vi "Remove UI without races.vi"(8 "error in":errorcluster, 11 "state in":T1) -> (0 "error out":errorcluster, 3 "state out":T1)   [LabVIEW 2013, in "Standard Editor.lvlib"]
uses:
  Standard Editor.lvlib
  Controls/StateCluster.ctl
  Configuration Editor/Classes/SystemConfigRepo/SystemConfigRepo.lvclass
  Configuration Editor/Classes/Systems/Systems.lvclass
  <vilib>/NI/Configuration Framework/Node/StandardEvents.ctl
  <vilib>/NI/Configuration Framework/Node/UserEventRef.ctl
  <vilib>/NI/Configuration Framework/Controls/EventCluster.ctl
  <vilib>/NI/Configuration Framework/Node/NodeChangeEvent.ctl
  <vilib>/NI/Configuration Framework/Node/NodeRef.ctl
  <vilib>/NI/Configuration Framework/Node/NISE_CEF_Node.lvclass
  <vilib>/NI/Configuration Framework/Node/CacheState.ctl
  <vilib>/NI/Configuration Framework/Node/RefreshUIEvent.ctl
  <vilib>/NI/Configuration Framework/Node/StopEvent.ctl
  <vilib>/NI/Configuration Framework/glyph manager/glyph manager.ctl
  <vilib>/picture/picture.llb/imagedata.ctl
  <vilib>/NI/AMC/Message Queue.ctl
  <vilib>/NI/AMC/Message.ctl
  <vilib>/NI/Tools/Keyed Array/KeyedArray.ctl
  <vilib>/event_ctls.llb/usereventprio.ctl
  <vilib>/NI/Configuration Framework/NISE_CEF_TreeControl.lvlib
  <vilib>/NI/Configuration Framework/glyph manager/glyph manager.lvlib
  <vilib>/NI/Tools/Keyed Array/Tools_KeyedArray.lvlib
  <vilib>/NI/AMC/AMC.lvlib
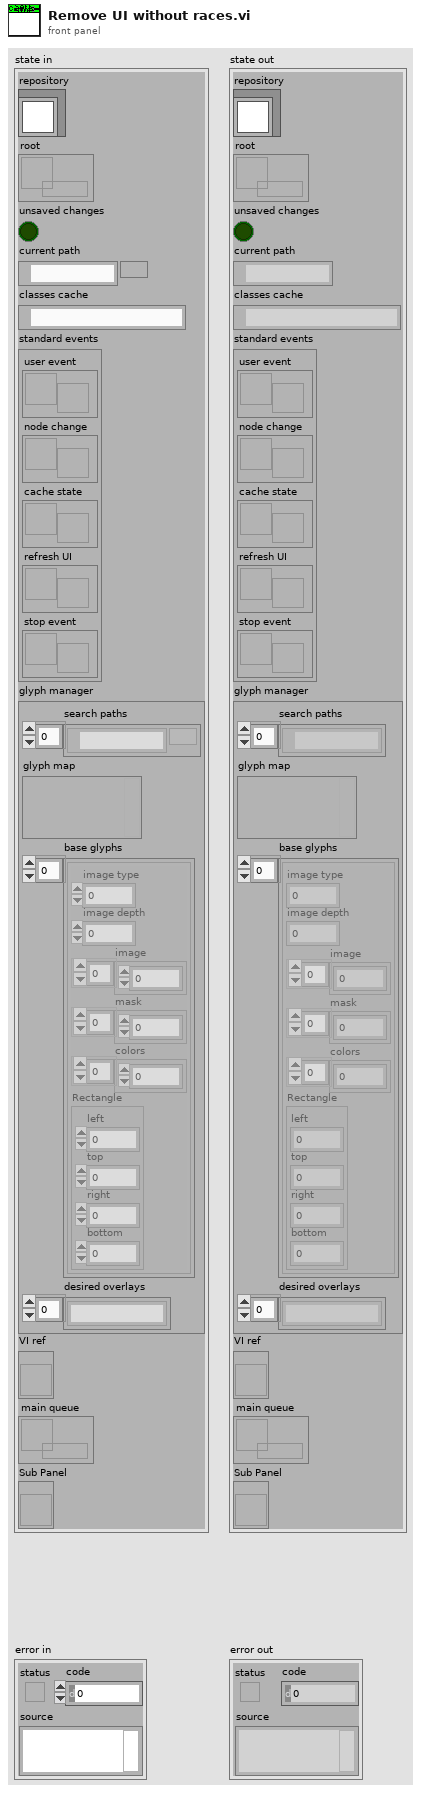
[diagram p1: front panel]
types:
  T1 = typedef "Standard Editor.lvlib/StateCluster.ctl" = cluster{"repository":refnum<class "SystemConfigRepo.lvclass">, "root":refnum<data-value>, "unsaved changes":bool, "current path":path, "classes cache":path, "standard events":T2, "glyph manager":T8, "VI ref":refnum<vi>, "main queue":T10, "Sub Panel":refnum<vi>}
  T2 = typedef "NISE_CEF_Node.lvclass/StandardEvents.ctl" = cluster{"user event":T3, "node change":T4, "cache state":T5, "refresh UI":T6, "stop event":T7}
  T3 = typedef "NISE_CEF_Node.lvclass/UserEventRef.ctl" = refnum<user-event>
  T4 = typedef "NISE_CEF_Node.lvclass/NodeChangeEvent.ctl" = refnum<user-event>
  T5 = typedef "NISE_CEF_Node.lvclass/CacheState.ctl" = refnum<user-event>
  T6 = typedef "NISE_CEF_Node.lvclass/RefreshUIEvent.ctl" = refnum<user-event>
  T7 = typedef "NISE_CEF_Node.lvclass/StopEvent.ctl" = refnum<user-event>
  T8 = typedef "glyph manager.lvlib/glyph manager.ctl" = cluster{"search paths":path[], "glyph map":variant, "base glyphs":T9[], "desired overlays":string[]}
  T9 = typedef "imagedata.ctl" = cluster{"image type":i32, "image depth":i32, "image":u8[], "mask":u8[], "colors":u32[], "Rectangle":cluster{"left":i16, "top":i16, "right":i16, "bottom":i16}}
  T10 = typedef "AMC.lvlib/Message Queue.ctl" = refnum<queue>
  T11 = typedef "usereventprio.ctl" = enum32{"high priority", "normal priority"}
  T12 = typedef "NISE_CEF_TreeControl.lvlib/EventCluster.ctl" = cluster{"command":string, "data":string}
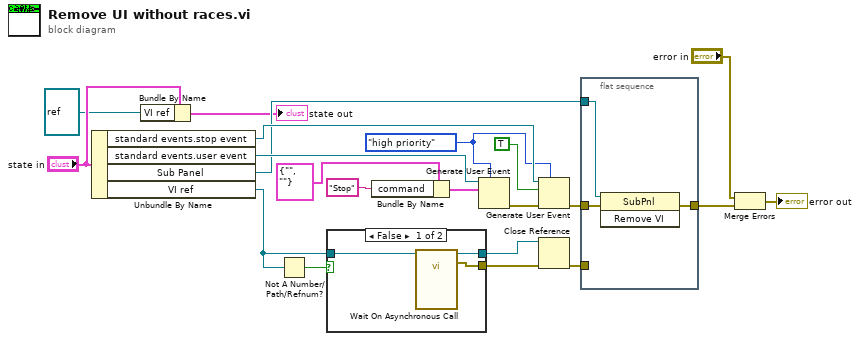
[diagram p0: block diagram]
diagram:
  w1 = usereventprio."high priority" ("priority (normal)")
  n1 = Unbundle By Name("state in") -> ("standard events.stop event"=w18:T7, "standard events.user event"=w19:T3, "Sub Panel"=w17:refnum<vi>, "VI ref"=w5:refnum<vi>)
  n2 = Bundle By Name(cluster="state in", "VI ref"=refnum<vi> refnum) -> (→"state out":T1)
  n3 = Not A Number/Path/Refnum?(number/path/refnum=w5) -> (NaN/Path/Refnum?=w6:bool)
  n4 = case shown="False" w6 {
    tunnel: w5 -> [w24 w25]
    tunnel: [w22 w25] -> w4
    tunnel: [w23 _] -> w3
    frame False {
      n5 = call-by-ref "Wait On Asynchronous Call"(reference=w24) -> (reference out=w22:refnum<vi>, error out=w23:errorcluster)  [unwired: 13 in]
    }
    frame True {
    }
  }
  n6 = Bundle By Name(cluster=T12 {"command"="", "data"=""} ("event data"), "command"="Stop") -> (w13:T12)
  n7 = Generate User Event(priority (normal)=w1, user event=w19, event data cluster=w13) -> (error out=w11:errorcluster)  [unwired: 1 in, 1 out]
  n8 = Generate User Event(priority (normal)=w1, user event=w18, event data cluster=TRUE ("event data"), error in=w11) -> (error out=w16:errorcluster)  [unwired: 1 out]
  n9 = Close Reference(reference=w4, error in (no error)=w3) -> (error out=w2:errorcluster)
  n10 = flat-sequence {
    tunnel: w17 -> [w28]
    tunnel: w16 -> [w27]
    tunnel: [w26] -> w15
    tunnel: w2 -> [_]
    frame #0 {
      n11 = invoke class="SubPnl" method="Remove VI"(reference=w28, error in=w27) -> (error out=w26:errorcluster)  [unwired: 1 in, 2 out]
    }
  }
  n12 = Merge Errors("error in", w15) -> (→"error out":errorcluster)
